vi "Initialize.vi"(8 "error in (no error)":errorcluster, 11 "EPOS4 Settings In":T1={"VISA resource name"="", "axis"={"keyHandle"=1, "nodeId"=1}, "Simulated?"=FALSE}) -> (0 "error out":errorcluster, 1 "Initialized":bool, 2 "No EPOS4 Connected":bool, 3 "EPOS4 Settings Out":T1={"VISA resource name"="", "axis"={"keyHandle"=1, "nodeId"=1}, "Simulated?"=FALSE})   [LabVIEW 2018, in "EPOS4.lvlib"]
uses:
  EPOS4.lvlib
  Controls/EPOS Communication Settings.ctl
panel:
  in  "position profile":T2={"profileVelocity"=1000, "profileAcceleration"=10000, "profileDeceleration"=10000}
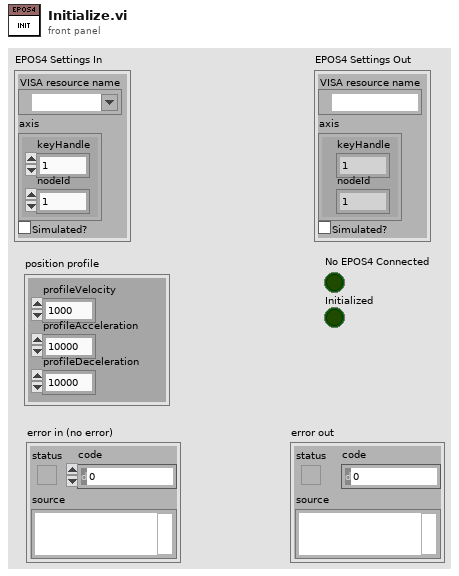
[diagram p1: front panel]
types:
  T1 = typedef "EPOS4.lvlib/EPOS Communication Settings.ctl" = cluster{"VISA resource name":refnum<visa-resource-name>, "axis":cluster{"keyHandle":u32, "nodeId":u16}, "Simulated?":bool}
  T2 = cluster{"profileVelocity":u32, "profileAcceleration":u32, "profileDeceleration":u32}
  T3 = cluster{"deviceName":string, "protocolStackName":string, "interfaceName":string, "portName":string, "baudrate":u32, "timeout":u32}
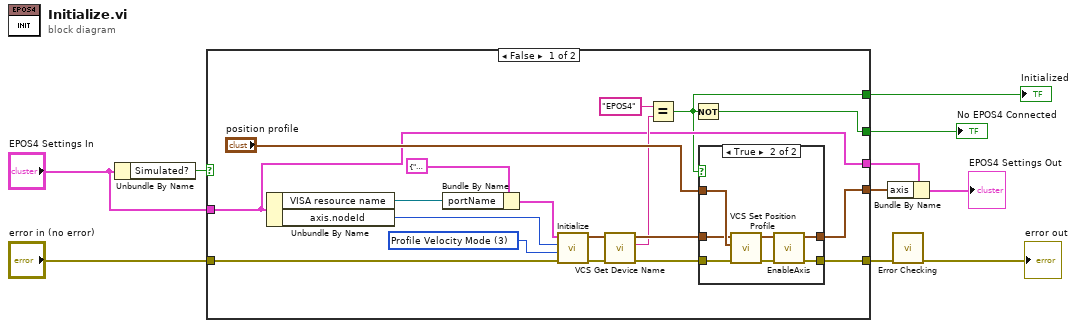
[diagram p0: block diagram]
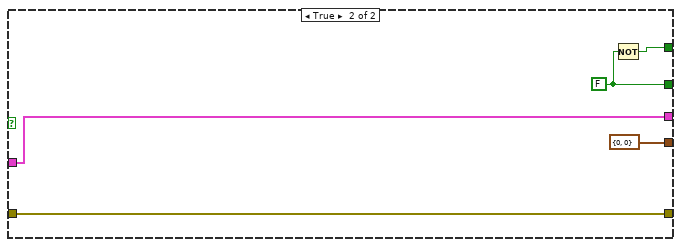
[diagram p3: hidden frame]
diagram:
  n1 = Unbundle By Name("EPOS4 Settings In") -> ("Simulated?"=w7:bool)
  n2 = case shown="False" w7 {
    tunnel: "EPOS4 Settings In" -> [w13 w39]
    tunnel: [w16 w42] -> w10
    tunnel: "error in (no error)" -> [w15 w42]
    tunnel: [w14 w40] -> w5
    tunnel: [w11 w41] -> w4
    tunnel: [w13 w39] -> w3
    tunnel: [w12 cluster{"keyHandle":u32, "nodeId":u16} {"keyHandle"=0, "nodeId"=0} ("axis out")] -> w1
    frame False {
      w24 = i8 3 items=["Profile Position Mode"=1, "Profile Velocity Mode"=3, "Homing Mode"=6, "Interpolated Position Mode"=7, "Position Mode"=-1, "Velocity Mode"=-2, "Current Mode"=-3, "Master Encoder Mode"=-5, "Step Direction Mode"=-6] ("modes of operations")
      n3 = Unbundle By Name(w13) -> ("VISA resource name"=w28:refnum<visa-resource-name>, "axis.nodeId"=w25:u16)
      n4 = Bundle By Name(cluster=T3 {"deviceName"="EPOS4", "protocolStackName"="MAXON SERIAL V2", "interfaceName"="RS232", "portName"="COM1", "baudrate"=115200, "timeout"=500} ("communication settings in"), "portName"=w28) -> (w26:T3)
      n5 = call "Initialize.vi"("error in (no error)"=w15, "modes of operations"=w24, "nodeId"=w25, "communication settings in"=w26) -> ("error out"=w17:errorcluster, "axis out"=w22:cluster{"keyHandle":u32, "nodeId":u16})  [unwired: 6 in]
      n6 = call "VCS Get Device Name.vi"("error in (no error)"=w17, "axis in"=w22) -> ("error out"=w18:errorcluster, "deviceName"=w19:string, "axis out"=w21:cluster{"keyHandle":u32, "nodeId":u16})  [unwired: 7 in]
      n7 = Equal?(x="EPOS4", y=w19) -> (x = y?=w11:bool)
      n8 = Not(x=w11) -> (.not. x?=w14:bool)
      n9 = case shown="True" w11 {
        tunnel: "position profile" -> [_ w37]
        tunnel: w21 -> [w29 w36]
        tunnel: w18 -> [w30 w35]
        tunnel: [w30 w32] -> w16
        tunnel: [w29 w31] -> w12
        frame False {
        }
        frame True {
          n10 = call "VCS Set Position Profile.vi"("error in (no error)"=w35, "position profile"=w37, "axis in"=w36) -> ("error out"=w33:errorcluster, "axis out"=w34:cluster{"keyHandle":u32, "nodeId":u16})  [unwired: 7 in]
          n11 = call "EnableAxis.vi"("error in (no error)"=w33, "axis in"=w34) -> ("error out"=w32:errorcluster, "axis out"=w31:cluster{"keyHandle":u32, "nodeId":u16})  [unwired: 4 in]
        }
      }
    }
    frame True {
      w40 = FALSE
      n12 = Not(x=w40) -> (.not. x?=w41:bool)
    }
  }
  "Initialized" <- w4
  "No EPOS4 Connected" <- w5
  n13 = Bundle By Name(cluster=w3, "axis"=w1) -> (→"EPOS4 Settings Out":T1)
  n14 = call "Error Checking.vi"("error in (no error)"=w10) -> ("error out"=→"error out":errorcluster)  [unwired: 8 in, 2 out]
